vi "MasterAquisitionFile_IOS_Optogenetics_Test.vi"() -> ()   [LabVIEW 2018]
uses:
  <vilib>/vision/driver/IMAQdx.llb/IMAQdx Acquisition Mode.ctl
  <vilib>/vision/driver/IMAQdx.llb/IMAQdx Camera Control Mode.ctl
  <vilib>/userdefined/High Color/IMAQdx.ctl
  <vilib>/vision/driver/IMAQdx.llb/IMAQdx Buffer Number Mode.ctl
  <vilib>/DAQmx/write.llb/DAQmx Write (Analog 1D DBL 1Chan NSamp).vi
  <vilib>/DAQmx/write.llb/DAQmx Write (Digital Bool 1Line 1Point).vi
  <vilib>/DAQmx/read.llb/DAQmx Read (Analog 1D Wfm NChan NSamp).vi
  <vilib>/DAQmx/write.llb/DAQmx Write (Digital 1D Bool 1Chan 1Samp).vi
  <vilib>/DAQmx/create/channels.llb/DAQmx Create Channel (DO-Digital Output).vi
  <vilib>/Waveform/DWDTOps.llb/DWDT Digital to Boolean Array.vi
  <vilib>/DAQmx/create/channels.llb/DAQmx Create Channel (AO-Voltage-Basic).vi
  <vilib>/DAQmx/create/channels.llb/DAQmx Create Channel (CO-Pulse Generation-Frequency).vi
  <vilib>/DAQmx/configure/timing.llb/DAQmx Timing (Implicit).vi
  <vilib>/DAQmx/create/channels.llb/DAQmx Create Channel (AI-Voltage-Basic).vi
  <vilib>/DAQmx/configure/timing.llb/DAQmx Timing (Sample Clock).vi
  <vilib>/DAQmx/configure/trigger.llb/DAQmx Start Trigger (Digital Edge).vi
  <vilib>/DAQmx/miscellaneous.llb/DAQmx Fill In Error Info.vi
  <vilib>/vision/driver/NI_Vision_Acquisition_Software.lvlib
  <resource>/objmgr/imaqdx.rc
  <resource>/objmgr/daqmx.rc
panel:
  out "LED":bool
  out "Auditory":bool
  out "RPad":bool
  out "LPad":bool
  out "Finished":bool
  in  "Solenoids":bool=TRUE
  in  "LED":bool=TRUE
  in  "Sol Stim Parameters":cluster{"Fs":dbl, "Samples":dbl}
  in  "LED Stim Parameters":cluster{"Fs":dbl, "Samples":dbl}
  in  "Sol Duty Cycle (%)":dbl=10.0
  in  "Sol Freq":dbl=1.0
  in  "Sol Dur (s)":dbl=1.0
  in  "LED Duty Cycle (%)":dbl=10.0
  in  "LED Freq":dbl=10.0
  in  "LED Dur (s)":dbl=2.0
  out "Stimulus Order":digitalwaveform[](graph)=[{"t0"=timestamp(0 s since 1904-01-01), "dt"=5e-05, "Y"={"transitions"=[], "data"=array18000000x1[18000000 elements]}}, {"t0"=timestamp(0 s since 1904-01-01), "dt"=5e-05, "Y"={"transitions"=[], "data"=array18000000x1[18000000 elements]}}, {"t0"=timestamp(0 s since 1904-01-01), "dt"=5e-05, "Y"={"transitions"=[], "data"=array18000000x1[18000000 elements]}}, {"t0"=timestamp(0 s since 1904-01-01), "dt"=5e-05, "Y"={"transitions"=[], "data"=array18000000x1[18000000 elements]}}]
  out "Solenoid Stim":digitalwaveform(graph)={"t0"=timestamp(0 s since 1904-01-01), "dt"=5e-05, "Y"={"transitions"=[], "data"=array20000x1[20000 elements]}}
  in  "Trial Offset (s)":dbl=15.0
  in  "Interstim (s)":dbl=30.0
  in  "Right Pad":dbl=1.0
  in  "Left Pad":dbl=1.0
  in  "Auditory":dbl=1.0
  in  "LED":dbl
  out "Dev2 Samples":i32
  out "Dev2 Analog":bool
  in  "Dev2 Analog Channels":string[](array[string])=["LD_BackScatter", "LD_Flow", "Opto_LED", "RPadSol", "AudSol", "Hippocampus", "EMG", "Cortical_RH"]
  out "?":T1(plugin-control)
  out "?":T1(plugin-control)
  out "?":T1(plugin-control)
  out "?":T1(plugin-control)
  in  "stop":bool
  out "CBV Cam":bool
  out "Pupil Cam":bool
  out "Whisk Cam":bool
  out "Web Cam":bool
  out "Dev1 Analog":bool
  out "Web Cam Fs":dbl(knob) scale=0.0..200.0
  out "CBV Cam":dbl(knob) scale=0.0..200.0
  out "Whisk Cam Fs":dbl(knob) scale=0.0..200.0
  out "Last Whisk\nBuffer 2":u32=574
  out "Pupil Cam Fs":dbl(knob) scale=0.0..200.0
  out "Dropped 2":u32(slide) caption="Pupil Cam" scale=0.0..99.0
  in  "Exposure Time (microsec)":string="10000"
  out "Dev1 Samples":i32
  in  "Dev1 Analog Channels":string[](array[string])=["Cortical_LH", "Force_Sensor", "LPadSol", "RPadSol", "AudSol", "Hippocampus", "EMG", "Cortical_RH"]
  in  "Analog Acquisition":cluster{"Analog Fs":u16}={"Analog Fs"=20000} {"Analog Fs" format="%0.0f"}
  in  "Sampling Rates":T2={"CBV Cam Fs"=30, "Whisk Cam Fs"=150, "Web Cam Fs"=15, "Pupil Cam Fs"=30}
  out "Notes Size":i32=7
  out "Notes Reversed":string[](array[string])=["Experimenter", "Animal ID", "Hemisphere", "Solenoid PSI", "Isoflurane time", "Session ID", "Amplifier Gain"]
  out "Notes Array":string[](array[string])=["Amplifier Gain", "Session ID", "Isoflurane time", "Solenoid PSI", "Hemisphere", "Animal ID", "Experimenter"]
  in  "Notes:":T3={"Experimenter"="Kevin", "Animal ID"="T155", "Hemisphere"="Both", "Solenoid PSI"="10", "Isoflurane time"="815", "Session ID"="Imaging Session Four", "Amplifier Gain"="10000", "LED power (mW)"="0"}
  in  "Target Path":path=path "D:/T155/Imaging Session 4 - 7 Nov. 2020" caption="Final Save Location"
  out "Dropped":u32(slide) caption="Whisk Cam" scale=0.0..999.0
  out "Filename":string="201105_15_03_37"
  out "CBV Camera":bool
  out "Time Elapsed (Min)":cluster{dbl, dbl}(slide)={15.0, 0.0} scale=0.0..15.0 scale format="%#_2g"
  in  "Time (min)":dbl(knob)=15.0 min=0.5 max=20.0 step=0.5 scale=0.0..20.0 scale format="%#_2g"
  in  "Temp Path":path=path "D:/LabVIEW Streamed Data" caption="Temporary Path for Streamed Data"
  out "Last CBV\nBuffer":i32=574
  out "Last Whisk\nBuffer":u32=2874
  # "Stimuli"
  # "LPAD"
  # "RPAD"
  # "AUD"
  # "LED"
  # "Ratio"
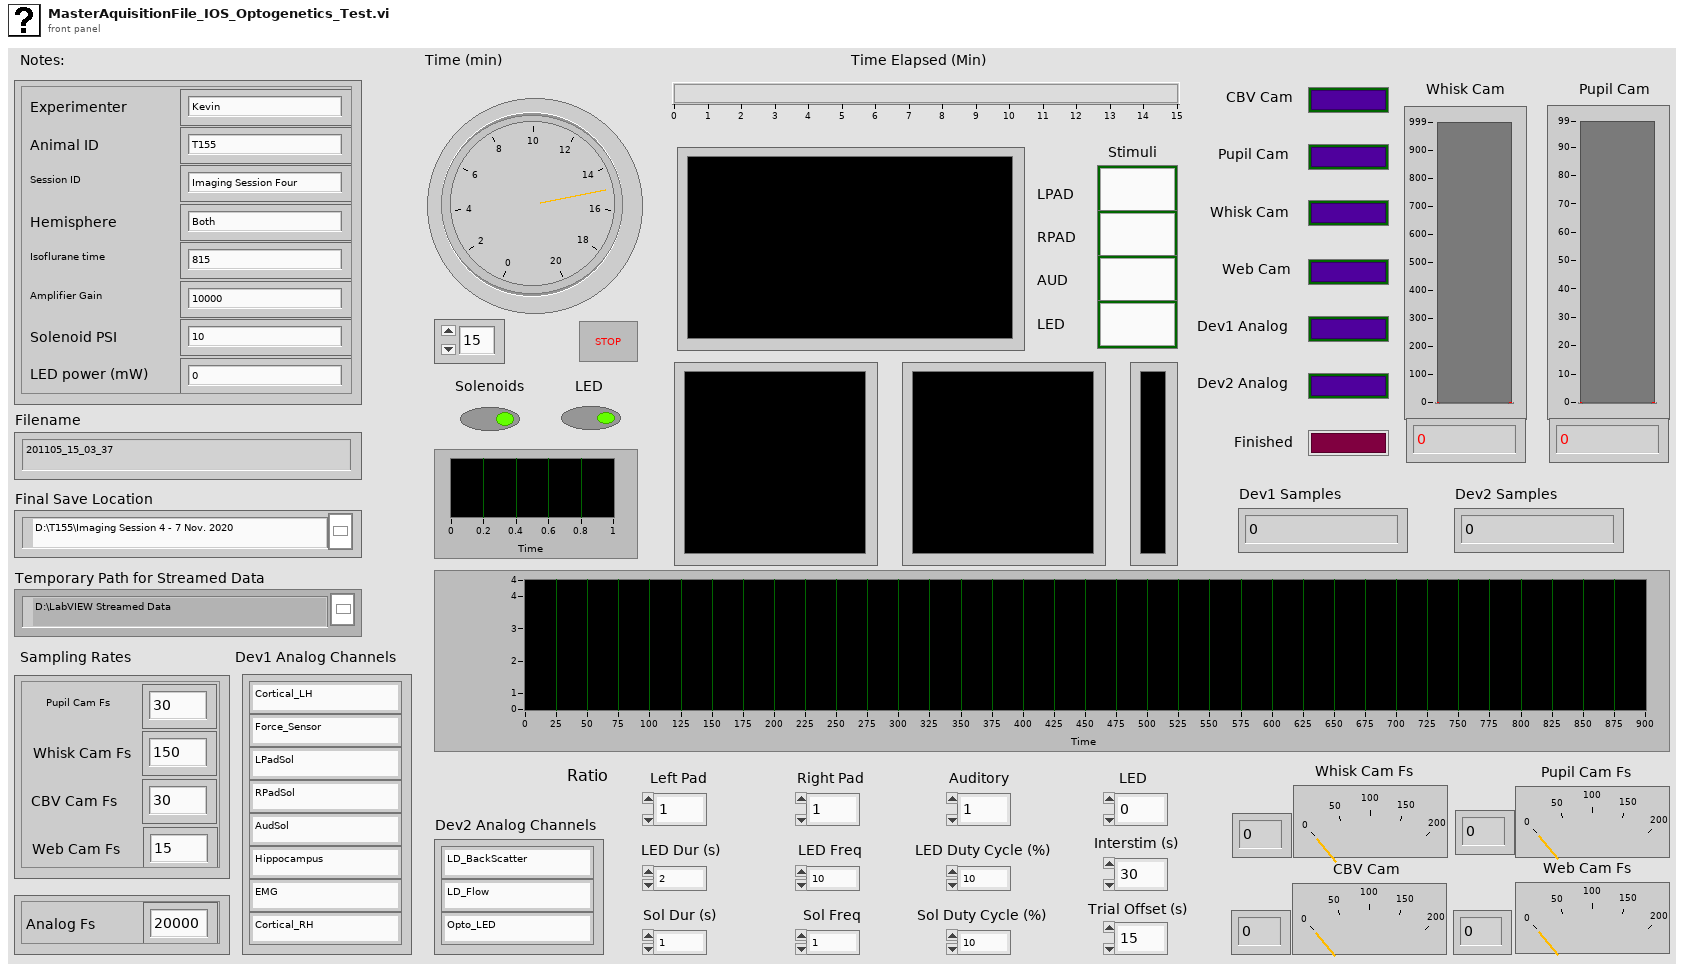
[diagram p1: front panel]
types:
  T1 = typedef "IMAQ Image.ctl" = refnum<image>
  T2 = cluster{"CBV Cam Fs":u16, "Whisk Cam Fs":u16, "Web Cam Fs":u16, "Pupil Cam Fs":u16}
  T3 = cluster{"Experimenter":string, "Animal ID":string, "Hemisphere":string, "Solenoid PSI":string, "Isoflurane time":string, "Session ID":string, "Amplifier Gain":string, "LED power (mW)":string}
  T4 = typedef "IMAQdx.ctl" = refnum<k21>
  T5 = enum16{"open", "open or create", "create or replace", "create", "open (read-only)"}
  T6 = enum16{"open", "replace", "create", "open or create", "replace or create", "replace or create with confirmation"}
  T7 = typedef "Image Type" = u32
  T8 = typedef "NI_Vision_Acquisition_Software.lvlib/IMAQdx Acquisition Mode.ctl" = enum32{"One Shot", "Continuous"}
  T9 = typedef "NI_Vision_Acquisition_Software.lvlib/IMAQdx Camera Control Mode.ctl" = enum32{"Controller", "Listener"}
  T10 = typedef "IMAQ AVI2 Refnum.ctl" = refnum<k20>
  T11 = enum16{"big-endian, network order", "native, host order", "little-endian"}
  T12 = typedef "NI_Vision_Acquisition_Software.lvlib/IMAQdx Buffer Number Mode.ctl" = enum32{"Next", "Last", "Buffer Number", "Every", "Last New"}
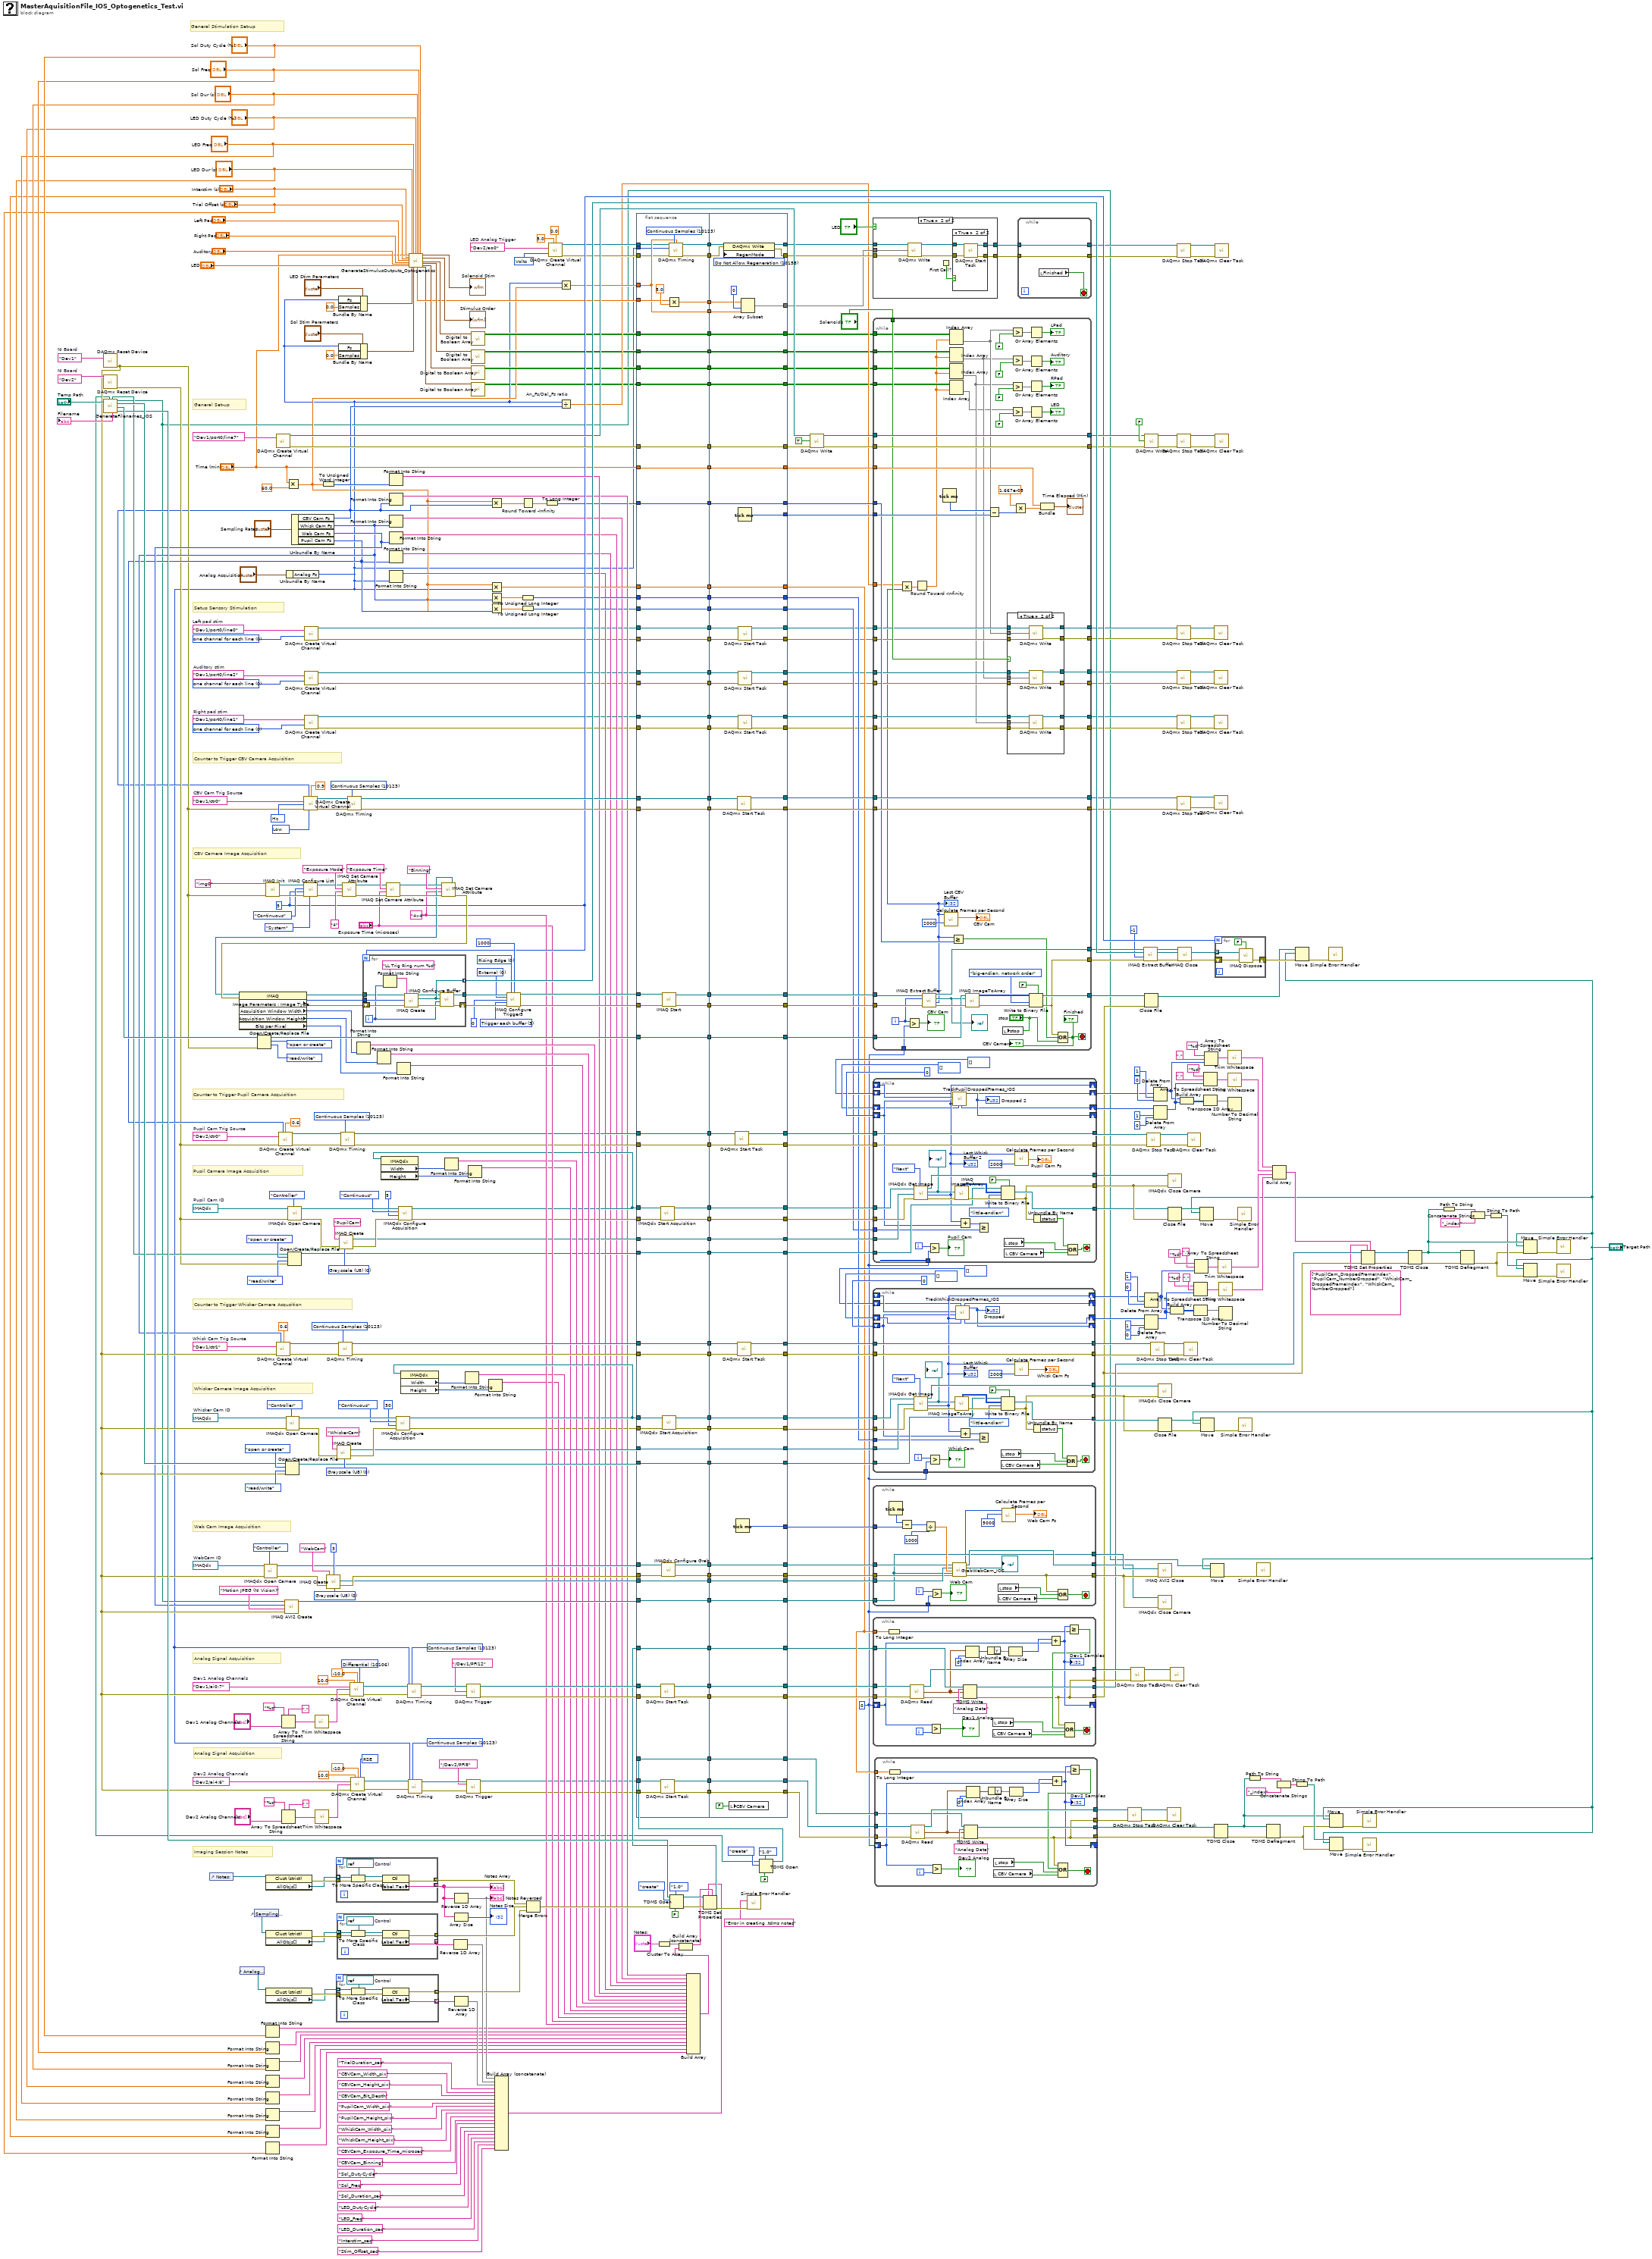
[diagram p0: block diagram]
diagram:
  w159 = tag "Dev2/ai4:6"  # Dev2 Analog Channels
  w357 = tag "Dev1/ai0:7"  # Dev1 Analog Channels
  w360 = T4 "cam0"  # WebCam ID
  w338 = T4 "cam1"  # Whisker Cam ID
  w532 = tag "Dev1/ctr1"  # Whisk Cam Trig Source
  w259 = T4 "cam2"  # Pupil Cam ID
  w264 = tag "Dev2/ctr0"  # Pupil Cam Trig Source
  w506 = tag "Dev1/ctr0"  # CBV Cam Trig Source
  w81 = tag "Dev1/port0/line1"  # Right pad stim
  w79 = tag "Dev1/port0/line0"  # Left pad stim
  w80 = tag "Dev1/port0/line2"  # Auditory stim
  w32 = 0 items=["one channel for each line", "one channel for all lines"] ("line grouping")
  w82 = 0 items=["one channel for each line", "one channel for all lines"] ("line grouping")
  w83 = 0 items=["one channel for each line", "one channel for all lines"] ("line grouping")
  w101 = 10348 items=["Volts"=10348, "From Custom Scale"=10065] ("units")
  w102 = tag "Dev2/ao0"  # LED Analog Trigger
  w163 = 10123 items=["Finite Samples"=10178, "Continuous Samples"=10123, "Hardware Timed Single Point"=12522] ("sample mode")
  w166 = 10083 items=["default"=-1, "RSE"=10083, "NRSE"=10078, "Differential"=10106, "Pseudodifferential"=12529] ("input terminal configuration")
  w182 = tag "Dev2"  # NI Board
  w260 = 10123 items=["Finite Samples"=10178, "Continuous Samples"=10123, "Hardware Timed Single Point"=12522] ("sample mode")
  w267 = T7 0 items=["Grayscale (U8)", "Grayscale (I16)", "Grayscale (SGL)", "Complex (CSG)", "RGB (U32)", "HSL (U32)", "RGB (U64)", "Grayscale (U16)"] ("Image Type")
  w249 = "4x4" ("Attribute Value")
  w118 = 0
  w439 = 10123 items=["Finite Samples"=10178, "Continuous Samples"=10123, "Hardware Timed Single Point"=12522] ("sample mode")
  w442 = 10106 items=["default"=-1, "RSE"=10083, "NRSE"=10078, "Differential"=10106, "Pseudodifferential"=12529] ("input terminal configuration")
  w493 = T7 0 items=["Grayscale (U8)", "Grayscale (I16)", "Grayscale (SGL)", "Complex (CSG)", "RGB (U32)", "HSL (U32)", "RGB (U64)", "Grayscale (U16)"] ("Image Type")
  w513 = u32 0 items=["Rising Edge", "Falling Edge"] ("Trigger Polarity")
  w516 = u32 0 items=["External"=0, "RTSI"=1, "ISO In"=2, "Scaled Encoder"=5] ("Trigger Type")
  w507 = tag "Dev1"  # NI Board
  w508 = 10123 items=["Finite Samples"=10178, "Continuous Samples"=10123, "Hardware Timed Single Point"=12522] ("sample mode")
  w511 = 10373 items=["Hz"=10373] ("units")
  w512 = 10214 items=["High"=10192, "Low"=10214] ("idle state")
  w278 = u32 5 ("Number of Buffers")
  w514 = u32 3 items=["Disabled", "Trigger start of acquisition", "Trigger start of each buffer list", "Trigger each buffer", "Trigger each line (linescan)", "Trigger end of acquisition"] ("Action")
  w528 = 10123 items=["Finite Samples"=10178, "Continuous Samples"=10123, "Hardware Timed Single Point"=12522] ("sample mode")
  w535 = T7 0 items=["Grayscale (U8)", "Grayscale (I16)", "Grayscale (SGL)", "Complex (CSG)", "RGB (U32)", "HSL (U32)", "RGB (U64)", "Grayscale (U16)"] ("Image Type")
  # "General Stimulation Set-up"
  # "Analog Signal Acquisition"
  # "General Set-up"
  # "Pupil Camera Image Acquisition"
  # "Counter to Trigger Pupil Camera Acquisition"
  # "Whisker Camera Image Acquisition"
  # "Imaging Session Notes"
  # "Setup Sensory Stimulation"
  # "CBV Camera Image Acquisition"
  # "Counter to Trigger CBV Camera Acquisition"
  # "Counter to Trigger Whisker Camera Acqusition"
  # "Web Cam Image Acquisition"
  # "Analog Signal Acquisition"
  n1 = call <vilib>:"DAQmx Reset Device.vi"("device in"=w507) -> ("error out"=w152:errorcluster)  [unwired: 14 in]
  n2 = call <vilib>:"DAQmx Reset Device.vi"("device in"=w182) -> ("error out"=w181:errorcluster)  [unwired: 14 in]
  n3 = call "GenerateFilenames_IOS.vi"("path"="Temp Path") -> ("TDMS Path"=w382:path, "Dalsa Path"=w500:path, "Basler Path"=w496:path, "WebCam Path"=w31:path, "Analog file name"=→"Filename":string, "Basler2 Path"=w258:path, "TDMS Path 2"=w120:path)  [unwired: 3 in, 1 out]
  n4 = control-ref of="Notes:"() -> (w387:refnum<vi>)
  n5 = control-ref of="Analog Acquisition"() -> (w365:refnum<vi>)
  n6 = control-ref of="Sampling Rates"() -> (w366:refnum<vi>)
  n7 = Open/Create/Replace File(file path (use dialog)=w500, error in=w152, operation (0:open)=T6."open or create", access (0:read/write)=enum16{"read/write", "read-only", "write-only"}."read/write") -> (refnum out=w443:refnum<file>)  [unwired: 2 in, 2 out]
  n8 = call <vilib>:"IMAQdx Open Camera.vi"("Camera Control Mode"=IMAQdx_Camera_Control_Mode."Controller", "error in"=w152, "Session In"=w360) -> ("error out"=w489:errorcluster, "Session Out"=w487:T4)  [unwired: 7 in]
  n9 = property class="Clust (strict)"(reference=w387) -> (error out=w390:errorcluster, "AllObjs[]"=w285:refnum<vi>[])  [unwired: 1 in, 1 out]
  n10 = property class="Clust (strict)"(reference=w366) -> (error out=w385:errorcluster, "AllObjs[]"=w286:refnum<vi>[])  [unwired: 1 in, 1 out]
  n11 = property class="Clust (strict)"(reference=w365) -> (error out=w364:errorcluster, "AllObjs[]"=w284:refnum<vi>[])  [unwired: 1 in, 1 out]
  n12 = call <vilib>:"IMAQ Init.vi"("error in (no error)"=w152, "Interface Name"="img0") -> ("error out"=w526:errorcluster, "IMAQ Session Out"=w527:refnum<k11>)  [unwired: 8 out]
  n13 = Format Into String("Sol Duty Cycle (%)") -> (resulting string=w20:string)  [unwired: 3 in, 1 out]
  n14 = Format Into String("Sol Freq") -> (resulting string=w19:string)  [unwired: 3 in, 1 out]
  n15 = Format Into String("Sol Dur (s)") -> (resulting string=w18:string)  [unwired: 3 in, 1 out]
  n16 = Format Into String("LED Duty Cycle (%)") -> (resulting string=w17:string)  [unwired: 3 in, 1 out]
  n17 = Format Into String("LED Freq") -> (resulting string=w16:string)  [unwired: 3 in, 1 out]
  n18 = Format Into String("LED Dur (s)") -> (resulting string=w15:string)  [unwired: 3 in, 1 out]
  n19 = Format Into String("Interstim (s)") -> (resulting string=w14:string)  [unwired: 3 in, 1 out]
  n20 = Format Into String("Trial Offset (s)") -> (resulting string=w13:string)  [unwired: 3 in, 1 out]
  n21 = call-poly <vilib>:"DAQmx Create Virtual Channel.vi"("lines"=tag "Dev1/port0/line7") -> ("task out"=w316:refnum<k21>, "error out"=w319:errorcluster)  [unwired: 13 in]
  n22 = Array To Spreadsheet String(delimiter (Tab)=",", array="Dev1 Analog Channels", 3:"%s" ("format string")) -> (spreadsheet string=w354:string)
  n23 = Array To Spreadsheet String(delimiter (Tab)=",", array="Dev2 Analog Channels", 3:"%s" ("format string")) -> (spreadsheet string=w156:string)
  n24 = Open/Create/Replace File(file path (use dialog)=w496, error in=w152, operation (0:open)=T6."open or create", access (0:read/write)=enum16{"read/write", "read-only", "write-only"}."read/write") -> (refnum out=w461:refnum<file>)  [unwired: 2 in, 2 out]
  n25 = Unbundle By Name("Analog Acquisition") -> ("Analog Fs"=w29:u16)
  n26 = call <vilib>:"IMAQdx Open Camera.vi"("Camera Control Mode"=IMAQdx_Camera_Control_Mode."Controller", "error in"=w152, "Session In"=w338) -> ("error out"=w538:errorcluster, "Session Out"=w541:T4)  [unwired: 7 in]
  n27 = Multiply(x="Time (min)", y=60.0) -> (x*y=w33:dbl)
  n28 = Open/Create/Replace File(file path (use dialog)=w258, error in=w181, operation (0:open)=T6."open or create", access (0:read/write)=enum16{"read/write", "read-only", "write-only"}."read/write") -> (refnum out=w239:refnum<file>)  [unwired: 2 in, 2 out]
  n29 = call <vilib>:"IMAQdx Open Camera.vi"("Camera Control Mode"=IMAQdx_Camera_Control_Mode."Controller", "error in"=w181, "Session In"=w259) -> ("error out"=w270:errorcluster, "Session Out"=w273:T4)  [unwired: 7 in]
  n30 = Unbundle By Name("Sampling Rates") -> ("CBV Cam Fs"=w84:u16, "Whisk Cam Fs"=w221:u16, "Web Cam Fs"=w359:u16, "Pupil Cam Fs"=w215:u16)
  n31 = call-poly <vilib>:"DAQmx Create Virtual Channel.vi"("frequency"=w221, "duty cycle"=0.6, "counter"=w532, "error in"=w152) -> ("task out"=w530:refnum<k21>, "error out"=w529:errorcluster)  [unwired: 10 in]
  n32 = call-poly <vilib>:"DAQmx Create Virtual Channel.vi"("frequency"=w215, "duty cycle"=0.6, "counter"=w264, "error in"=w181) -> ("task out"=w262:refnum<k21>, "error out"=w261:errorcluster)  [unwired: 10 in]
  n33 = call "IMAQ AVI2 Create"("error in (no error)"=w152, "Codec"="Motion JPEG (NI Vision)", "Frames Per Second"=w359, "AVI Path"=w31) -> ("AVI Refnum"=w479:T10)  [unwired: 6 in, 1 out]
  n34 = call-poly <vilib>:"DAQmx Create Virtual Channel.vi"("frequency"=w84, "duty cycle"=0.9, "counter"=w506, "units"=w511, "error in"=w152, "idle state"=w512) -> ("task out"=w510:refnum<k21>, "error out"=w509:errorcluster)  [unwired: 8 in]
  n35 = call <vilib>:"IMAQ Configure List.vi"("Memory Location"=enum16{"System", "Onboard"}."System", "error in (no error)"=w526, "Number of buffers"=w278, "Continuous?"=enum16{"One-Shot", "Continuous"}."Continuous" ("Continuous ?"), "IMAQ Session In"=w527) -> ("error out"=w299:errorcluster, "IMAQ Session Out"=w295:refnum<k11>)  [unwired: 1 in, 4 out]
  n36 = call-poly <vilib>:"DAQmx Create Virtual Channel.vi"("lines"=w79, "line grouping"=w32) -> ("task out"=w60:refnum<k21>, "error out"=w58:errorcluster)  [unwired: 12 in]
  n37 = call-poly <vilib>:"DAQmx Create Virtual Channel.vi"("lines"=w80, "line grouping"=w82) -> ("task out"=w56:refnum<k21>, "error out"=w54:errorcluster)  [unwired: 12 in]
  n38 = call-poly <vilib>:"DAQmx Create Virtual Channel.vi"("lines"=w81, "line grouping"=w83) -> ("task out"=w52:refnum<k21>, "error out"=w50:errorcluster)  [unwired: 12 in]
  n39 = call <vilib>:"Trim Whitespace.vi"("string"=w354) -> ("trimmed string"=w353:string)  [unwired: 1 in]
  n40 = call <vilib>:"Trim Whitespace.vi"("string"=w156) -> ("trimmed string"=w155:string)  [unwired: 1 in]
  n41 = To Unsigned Word Integer(number=w33) -> (unsigned 16bit integer=w349:u16)
  n42 = call "IMAQ Create"("Border Size"=3, "Image Name"="WebCam", "Image Type"=w493, "error in (no error)"=w489) -> ("New Image"=w486:T1, "error out"=w488:errorcluster)  [unwired: 1 in]
  n43 = for {
    tunnel: [w547] -> w389 mode=indexing
    tunnel: w390 -> [w546]
    tunnel: [w544] -> w373 mode=indexing
    tunnel: w285 -> [w543] mode=indexing
    w548 = refnum<vi> refnum  # Control
    n44 = To More Specific Class(target class=w548, reference=w543, error in=w546) -> (specific class reference=w549:refnum<vi>, error out=w545:errorcluster)
    n45 = property class="Ctl"(reference=w549, error in=w545) -> (error out=w544:errorcluster, "Label.Text"=w547:string)  [unwired: 1 out]
  }
  "Notes Array" <- w389
  n46 = for {
    tunnel: [w554] -> w362 mode=indexing
    tunnel: w364 -> [w553]
    tunnel: [w551] -> w363 mode=indexing
    tunnel: w284 -> [w550] mode=indexing
    w555 = refnum<vi> refnum  # Control
    n47 = To More Specific Class(target class=w555, reference=w550, error in=w553) -> (specific class reference=w556:refnum<vi>, error out=w552:errorcluster)
    n48 = property class="Ctl"(reference=w556, error in=w552) -> (error out=w551:errorcluster, "Label.Text"=w554:string)  [unwired: 1 out]
  }
  n49 = call "IMAQ Create"("Image Name"="WhiskerCam", "Image Type"=w535, "error in (no error)"=w538) -> ("New Image"=w336:T1, "error out"=w536:errorcluster)  [unwired: 2 in]
  n50 = for {
    tunnel: [w561] -> w386 mode=indexing
    tunnel: w385 -> [w560]
    tunnel: [w558] -> w372 mode=indexing
    tunnel: w286 -> [w557] mode=indexing
    w562 = refnum<vi> refnum  # Control
    n51 = To More Specific Class(target class=w562, reference=w557, error in=w560) -> (specific class reference=w563:refnum<vi>, error out=w559:errorcluster)
    n52 = property class="Ctl"(reference=w563, error in=w559) -> (error out=w558:errorcluster, "Label.Text"=w561:string)  [unwired: 1 out]
  }
  n53 = Bundle By Name(cluster="LED Stim Parameters", "Fs"=w29, "Samples"=0.0) -> (w107:cluster{"Fs":dbl, "Samples":dbl})
  n54 = Bundle By Name(cluster="Sol Stim Parameters", "Fs"=w29, "Samples"=0.0) -> (w108:cluster{"Fs":dbl, "Samples":dbl})
  n55 = call-poly <vilib>:"DAQmx Timing.vi"("task/channels in"=w530, "sample mode"=w528, "error in"=w529) -> ("task out"=w424:refnum<k21>, "error out"=w422:errorcluster)  [unwired: 11 in]
  n56 = call "IMAQ Create"("Image Name"="PupilCam", "Image Type"=w267, "error in (no error)"=w270) -> ("New Image"=w224:T1, "error out"=w268:errorcluster)  [unwired: 2 in]
  n57 = call-poly <vilib>:"DAQmx Timing.vi"("task/channels in"=w262, "sample mode"=w260, "error in"=w261) -> ("task out"=w237:refnum<k21>, "error out"=w235:errorcluster)  [unwired: 11 in]
  n58 = call <vilib>:"IMAQ Set Camera Attribute.vi"("error in (no error)"=w299, "Attribute Value"="4", "Camera Attribute"="Exposure Mode", "IMAQ Session In"=w295) -> ("error out"=w298:errorcluster, "IMAQ Session Out"=w294:refnum<k11>)  [unwired: 4 in]
  n59 = call-poly <vilib>:"DAQmx Timing.vi"("task/channels in"=w510, "sample mode"=w508, "error in"=w509) -> ("task out"=w428:refnum<k21>, "error out"=w426:errorcluster)  [unwired: 11 in]
  n60 = call-poly <vilib>:"DAQmx Create Virtual Channel.vi"("maximum value"=10.0, "minimum value"=-10.0, "input terminal configuration"=w442, "physical channels"=w357, "name to assign"=w353, "error in"=w152) -> ("task out"=w441:refnum<k21>, "error out"=w440:errorcluster)  [unwired: 8 in]
  n61 = call-poly <vilib>:"DAQmx Create Virtual Channel.vi"("maximum value"=10.0, "minimum value"=-10.0, "input terminal configuration"=w166, "physical channels"=w159, "name to assign"=w155, "error in"=w152) -> ("task out"=w165:refnum<k21>, "error out"=w164:errorcluster)  [unwired: 8 in]
  n62 = call <vilib>:"IMAQ Set Camera Attribute.vi"("error in (no error)"=w298, "Attribute Value"="Exposure Time (microsec)", "Camera Attribute"="Exposure Time", "IMAQ Session In"=w294) -> ("error out"=w297:errorcluster, "IMAQ Session Out"=w293:refnum<k11>)  [unwired: 4 in]
  n63 = Format Into String(w349) -> (resulting string=w351:string)  [unwired: 3 in, 1 out]
  n64 = Format Into String(w84) -> (resulting string=w219:string)  [unwired: 3 in, 1 out]
  n65 = Format Into String(w221) -> (resulting string=w218:string)  [unwired: 3 in, 1 out]
  n66 = Format Into String(w359) -> (resulting string=w217:string)  [unwired: 3 in, 1 out]
  n67 = Format Into String(w215) -> (resulting string=w168:string)  [unwired: 3 in, 1 out]
  n68 = Format Into String(w29) -> (resulting string=w167:string)  [unwired: 3 in, 1 out]
  n69 = call <vilib>:"IMAQdx Configure Acquisition.vi"("error in"=w536, "Number of Buffers"=u32 50, "Continuous?"=IMAQdx_Acquisition_Mode."Continuous", "Session In"=w541) -> ("error out"=w183:errorcluster, "Session Out"=w337:T4)  [unwired: 6 in]
  n70 = call <vilib>:"IMAQdx Configure Acquisition.vi"("error in"=w268, "Number of Buffers"=u32 5, "Continuous?"=IMAQdx_Acquisition_Mode."Continuous", "Session In"=w273) -> ("error out"=w241:errorcluster, "Session Out"=w225:T4)  [unwired: 6 in]
  n71 = property class="IMAQdx"(reference=w225) -> ("Width"=w257:u32, "Height"=w256:u32)  [unwired: 1 in, 2 out]
  n72 = property class="IMAQdx"(reference=w337) -> ("Width"=w348:u32, "Height"=w347:u32)  [unwired: 1 in, 2 out]
  n73 = call-poly <vilib>:"DAQmx Timing.vi"("task/channels in"=w441, "sample mode"=w439, "rate"=w29, "error in"=w440) -> ("task out"=w282:refnum<k21>, "error out"=w438:errorcluster)  [unwired: 10 in]
  n74 = call-poly <vilib>:"DAQmx Timing.vi"("task/channels in"=w165, "sample mode"=w163, "rate"=w29, "error in"=w164) -> ("task out"=w153:refnum<k21>, "error out"=w162:errorcluster)  [unwired: 10 in]
  n75 = call "GenerateStimulusOutputs_Optogenetics.vi"("Trial duration (min)"="Time (min)", "Rest duration(s)"="Interstim (s)", "trial offset (s)"="Trial Offset (s)", "Left Pad"="Left Pad", "Right Pad"="Right Pad", "Auditory"="Auditory", "LED"="LED", "LED Stim Duration (s)"="LED Dur (s)", "LED Stim Parameters"=w107, "LED Frequency"="LED Freq", "Sol Stim Parameters"=w108, "LED duty cycle (%)"="LED Duty Cycle (%)", "Sol Stim Duration (s)"="Sol Dur (s)", "Sol Frequency"="Sol Freq", "Sol Duty Cycle (%)"="Sol Duty Cycle (%)") -> ("Double LED Out"=w95:dbl[], "Solenoid Stim Waveforms"=→"Solenoid Stim":digitalwaveform, "Stimulus Digital Outputs"=→"Stimulus Order":digitalwaveform[], "Left Pad Out"=w113:digitalwaveform, "Auditory Out"=w112:digitalwaveform, "Right Pad Out"=w111:digitalwaveform, "LED Out"=w2:digitalwaveform)  [unwired: 6 in]
  n76 = call <vilib>:"IMAQ Set Camera Attribute.vi"("error in (no error)"=w297, "Attribute Value"=w249, "Camera Attribute"="Binning", "IMAQ Session In"=w293) -> ("error out"=w296:errorcluster, "IMAQ Session Out"=w292:refnum<k11>)  [unwired: 4 in]
  n77 = property class="IMAQ"(reference=w292, error in=w296) -> (reference out=w306:refnum<k11>, error out=w305:errorcluster, "Image Parameters : Image Type"=w522:u32, "Acquisition Window Width"=w346:u32, "Acquisition Window Height"=w345:u32, "Bits per Pixel"=w344:u32)
  n78 = Format Into String(w346) -> (resulting string=w343:string)  [unwired: 3 in, 1 out]
  n79 = for {
    N: w278 -> [_]
    tunnel: [w573] -> w518
    tunnel: w522 -> [w571]
    shift-right: [w572] -> w517
    shift-left: w305 -> [w570]
    tunnel: [w565] -> w519 mode=indexing
    tunnel: w306 -> [w564]
    i -> [w566]
    n80 = Format Into String(format string="LL Trig Ring num %d", w566) -> (resulting string=w568:string)  [unwired: 2 in, 1 out]
    n81 = call "IMAQ Create"("Image Name"=w568, "Image Type"=w571, "error in (no error)"=w570) -> ("New Image"=w565:T1, "error out"=w569:errorcluster)  [unwired: 1 in, 1 out]
    n82 = call <vilib>:"IMAQ Configure Buffer.vi"("error in (no error)"=w569, "Buffer Number"=w566, "Image In"=w565, "IMAQ Session In"=w564) -> ("error out"=w572:errorcluster, "IMAQ Session Out"=w573:refnum<k11>)  [unwired: 2 in, 4 out]
  }
  n83 = Format Into String(w345) -> (resulting string=w279:string)  [unwired: 3 in, 1 out]
  n84 = Format Into String(w344) -> (resulting string=w342:string)  [unwired: 3 in, 1 out]
  n85 = Format Into String(w257) -> (resulting string=w244:string)  [unwired: 3 in, 1 out]
  n86 = Reverse 1D Array(array=w386) -> (reversed array=w376:string[])
  n87 = Reverse 1D Array(array=w389) -> (reversed array=w283:string[])
  "Notes Reversed" <- w283
  n88 = Array Size(array=w389) -> (size(s)=→"Notes Size":i32)
  n89 = Reverse 1D Array(array=w362) -> (reversed array=w361:string[])
  n90 = Format Into String(w348) -> (resulting string=w246:string)  [unwired: 3 in, 1 out]
  n91 = call-poly <vilib>:"DAQmx Trigger.vi"("task/channels in"=w282, "source"=tag "/Dev1/PFI12", "error in"=w438) -> ("task out"=w437:refnum<k21>, "error out"=w436:errorcluster)  [unwired: 11 in]
  n92 = call-poly <vilib>:"DAQmx Trigger.vi"("task/channels in"=w153, "source"=tag "/Dev2/PFI8", "error in"=w162) -> ("task out"=w151:refnum<k21>, "error out"=w150:errorcluster)  [unwired: 11 in]
  n93 = Format Into String(w256) -> (resulting string=w245:string)  [unwired: 3 in, 1 out]
  n94 = call-poly <vilib>:"Digital to Boolean Array.vi"("digital waveform"=w113) -> ("boolean array"=w46:bool[][])  [unwired: 9 in, 1 out]
  n95 = call-poly <vilib>:"Digital to Boolean Array.vi"("digital waveform"=w112) -> ("boolean array"=w43:bool[][])  [unwired: 9 in, 1 out]
  n96 = call-poly <vilib>:"Digital to Boolean Array.vi"("digital waveform"=w111) -> ("boolean array"=w40:bool[][])  [unwired: 9 in, 1 out]
  n97 = call-poly <vilib>:"Digital to Boolean Array.vi"("digital waveform"=w2) -> ("boolean array"=w1:bool[][])  [unwired: 9 in, 1 out]
  n98 = Format Into String(w347) -> (resulting string=w247:string)  [unwired: 3 in, 1 out]
  n99 = Multiply(x=w33, y=w84) -> (x*y=w498:dbl)
  n100 = Multiply(x=w33, y=w29) -> (x*y=w325:dbl)
  n101 = Multiply(x=w221, y=w33) -> (x*y=w280:dbl)
  n102 = Multiply(x=w215, y=w33) -> (x*y=w220:dbl)
  n103 = Build Array (concatenate)(w283, w376, w361, "TrialDuration_sec", "CBVCam_Width_pix", "CBVCam_Height_pix", "CBVCam_Bit_Depth", "PupilCam_Width_pix", "PupilCam_Height_pix", "WhiskCam_Width_pix", "WhiskCam_Height_pix", "CBVCam_Exposure_Time_microsec" ("element"), "CBVCam_Binning" ("element"), "Sol_DutyCycle", "Sol_Freq", "Sol_Duration_sec", "LED_DutyCycle", "LED_Freq", "LED_Duration_sec", "Interstim_sec", "Stim_Offset_sec") -> (w275:string[])
  n104 = call <vilib>:"IMAQ Configure Trigger3.vi"("IMAQ Session In"=w518, "Polarity"=w513, "Frame timeout (ms)"=u32 1000 ("Frame Timeout (ms)"), "Type"=w516, "Line Number"=u32 0 ("Trigger Line Number"), "Action"=w514, "error in (no error)"=w517) -> ("IMAQ Session Out"=w460:refnum<k11>, "error out"=w459:errorcluster)  [unwired: 2 in, 5 out]
  n105 = To Unsigned Long Integer(number=w280) -> (unsigned 32bit integer=w323:u32)
  n106 = To Unsigned Long Integer(number=w220) -> (unsigned 32bit integer=w216:u32)
  n107 = Round Toward -Infinity(1:w498) -> (0:w497:dbl)
  n108 = Merge Errors(w373, w372, w363) -> (w371:errorcluster)
  n109 = To Long Integer(number=w497) -> (32bit integer=w184:i32)
  n110 = call-poly <vilib>:"DAQmx Create Virtual Channel.vi"("maximum value"=5.0, "minimum value"=0.0, "physical channels"=w102, "units"=w101) -> ("task out"=w91:refnum<k21>, "error out"=w88:errorcluster)  [unwired: 10 in]
  n111 = Multiply(x=w29, y=w33) -> (x*y=w93:dbl)
  n112 = Divide "An_Fs/Dal_Fs ratio"(x=w29, y=w84) -> (x/y=w47:dbl)
  n113 = flat-sequence {
    tunnel: w488 -> [w638]
    tunnel: w487 -> [w637]
    tunnel: w486 -> [w636]
    tunnel: [w636] -> w485
    tunnel: [w635] -> w483
    tunnel: [w634] -> w481
    tunnel: w479 -> [w633]
    tunnel: [w633] -> w478
    tunnel: w337 -> [w632]
    tunnel: w183 -> [w631]
    tunnel: [w630] -> w468
    tunnel: [w629] -> w466
    tunnel: [w628] -> w464
    tunnel: w336 -> [w628]
    tunnel: [w627] -> w462
    tunnel: w461 -> [w627]
    tunnel: w460 -> [w626]
    tunnel: w459 -> [w625]
    tunnel: [w624] -> w457
    tunnel: [w623] -> w455
    tunnel: w184 -> [w622]
    tunnel: [w622] -> w449
    tunnel: "Time (min)" -> [w621]
    tunnel: [w621] -> w446
    tunnel: [w620] -> w444
    tunnel: w443 -> [w620]
    tunnel: w437 -> [w619]
    tunnel: w436 -> [w618]
    tunnel: [w617] -> w435
    tunnel: [w616] -> w434
    tunnel: [w615] -> w430
    tunnel: w374 -> [w615]
    tunnel: w428 -> [w614]
    tunnel: [w614] -> w427
    tunnel: w426 -> [w613]
    tunnel: [w613] -> w425
    tunnel: w424 -> [w612]
    tunnel: [w612] -> w423
    tunnel: w422 -> [w611]
    tunnel: [w611] -> w421
    tunnel: w325 -> [w610]
    tunnel: [w610] -> w324
    tunnel: w323 -> [w609]
    tunnel: [w609] -> w322
    tunnel: w319 -> [w608]
    tunnel: [w608] -> w318
    tunnel: [w601] -> w243
    tunnel: w225 -> [w602]
    tunnel: [w599] -> w242
    tunnel: w241 -> [w600]
    tunnel: [w607] -> w240
    tunnel: w239 -> [w607]
    tunnel: [w606] -> w238
    tunnel: w237 -> [w606]
    tunnel: [w605] -> w236
    tunnel: w235 -> [w605]
    tunnel: w224 -> [w604]
    tunnel: [w604] -> w223
    tunnel: w216 -> [w603]
    tunnel: [w603] -> w214
    tunnel: w151 -> [w598]
    tunnel: w150 -> [w597]
    tunnel: [w596] -> w149
    tunnel: [w595] -> w148
    tunnel: w123 -> [w594]
    tunnel: [w594] -> w122
    tunnel: w95 -> [w591]
    tunnel: [w590] -> w94
    tunnel: w93 -> [w589]
    tunnel: [w589] -> w92
    tunnel: w91 -> [w588]
    tunnel: [w587] -> w90
    tunnel: [w586] -> w89
    tunnel: w88 -> [w585]
    tunnel: w29 -> [w584]
    tunnel: w60 -> [w583]
    tunnel: [w583] -> w59
    tunnel: w58 -> [w582]
    tunnel: [w582] -> w57
    tunnel: w56 -> [w581]
    tunnel: [w581] -> w55
    tunnel: w54 -> [w580]
    tunnel: [w580] -> w53
    tunnel: w52 -> [w579]
    tunnel: [w579] -> w51
    tunnel: w50 -> [w578]
    tunnel: [w578] -> w49
    tunnel: w46 -> [w577]
    tunnel: [w577] -> w45
    tunnel: w43 -> [w576]
    tunnel: [w576] -> w42
    tunnel: w40 -> [w575]
    tunnel: [w575] -> w39
    tunnel: w1 -> [w574]
    tunnel: [w574] -> w4
    tunnel: [w705] -> w490
    tunnel: w485 -> [w704]
    tunnel: [w704] -> w484
    tunnel: w483 -> [w703]
    tunnel: [w703] -> w482
    tunnel: w481 -> [w702]
    tunnel: [w702] -> w480
    tunnel: w478 -> [w701]
    tunnel: [w701] -> w477
    tunnel: [w683] -> w474
    tunnel: [w682] -> w472
    tunnel: [w700] -> w469
    tunnel: w468 -> [w700]
    tunnel: [w699] -> w467
    tunnel: w466 -> [w699]
    tunnel: [w698] -> w465
    tunnel: w464 -> [w698]
    tunnel: [w697] -> w463
    tunnel: w462 -> [w697]
    tunnel: [w696] -> w458
    tunnel: w457 -> [w696]
    tunnel: [w695] -> w456
    tunnel: w455 -> [w695]
    tunnel: [w687] -> w453
    tunnel: [w686] -> w451
    tunnel: [w694] -> w450
    tunnel: w449 -> [w693]
    tunnel: [w693] -> w448
    tunnel: [w692] -> w447
    tunnel: w446 -> [w692]
    tunnel: [w691] -> w445
    tunnel: w444 -> [w691]
    tunnel: [w690] -> w432
    tunnel: w435 -> [w690]
    tunnel: [w689] -> w433
    tunnel: w434 -> [w689]
    tunnel: [w688] -> w146
    tunnel: w430 -> [w688]
    tunnel: w427 -> [w685]
    tunnel: w425 -> [w684]
    tunnel: w423 -> [w681]
    tunnel: w421 -> [w680]
    tunnel: w324 -> [w679]
    tunnel: [w679] -> w147
    tunnel: w322 -> [w678]
    tunnel: [w678] -> w213
    tunnel: w318 -> [w677]
    tunnel: [w677] -> w317
    tunnel: w243 -> [w675]
    tunnel: w242 -> [w674]
    tunnel: w240 -> [w673]
    tunnel: w238 -> [w670]
    tunnel: w236 -> [w669]
    tunnel: [w667] -> w231
    tunnel: [w668] -> w230
    tunnel: [w675] -> w229
    tunnel: [w674] -> w228
    tunnel: [w673] -> w227
    tunnel: [w672] -> w222
    tunnel: w223 -> [w672]
    tunnel: [w671] -> w212
    tunnel: w214 -> [w671]
    tunnel: [w666] -> w144
    tunnel: w149 -> [w666]
    tunnel: [w665] -> w145
    tunnel: w148 -> [w665]
    tunnel: [w664] -> w121
    tunnel: w122 -> [w664]
    tunnel: w94 -> [w661]
    tunnel: w92 -> [w660]
    tunnel: w90 -> [w659]
    tunnel: w89 -> [w658]
    tunnel: [w657] -> w87
    tunnel: [w656] -> w86
    tunnel: [w655] -> w85
    tunnel: [w654] -> w66
    tunnel: [w653] -> w65
    tunnel: [w652] -> w64
    tunnel: [w651] -> w63
    tunnel: [w650] -> w62
    tunnel: [w649] -> w61
    tunnel: w59 -> [w648]
    tunnel: w57 -> [w647]
    tunnel: w55 -> [w646]
    tunnel: w53 -> [w645]
    tunnel: w51 -> [w644]
    tunnel: w49 -> [w643]
    tunnel: w45 -> [w642]
    tunnel: [w642] -> w44
    tunnel: w42 -> [w641]
    tunnel: [w641] -> w41
    tunnel: w39 -> [w640]
    tunnel: [w640] -> w38
    tunnel: w4 -> [w639]
    tunnel: [w639] -> w3
    frame #0 {
      w593 = 10123 items=["Finite Samples"=10178, "Continuous Samples"=10123, "Hardware Timed Single Point"=12522] ("sample mode")
      n114 = call <vilib>:"IMAQdx Start Acquisition.vi"("error in"=w600, "Session In"=w602) -> ("error out"=w599:errorcluster, "Session Out"=w601:T4)  [unwired: 8 in]
      n115 = call <vilib>:"DAQmx Start Task.vi"("task/channels in"=w619, "error in"=w618) -> ("task out"=w617:refnum<k21>, "error out"=w616:errorcluster)  [unwired: 12 in]
      n116 = call <vilib>:"DAQmx Start Task.vi"("task/channels in"=w598, "error in"=w597) -> ("task out"=w595:refnum<k21>, "error out"=w596:errorcluster)  [unwired: 12 in]
      n117 = call <vilib>:"IMAQdx Configure Grab.vi"("error in"=w638, "Session In"=w637) -> ("error out"=w634:errorcluster, "Session Out"=w635:T4)  [unwired: 8 in]
      n118 = call <vilib>:"IMAQ Start.vi"("error in (no error)"=w625, "IMAQ Session In"=w626) -> ("error out"=w623:errorcluster, "IMAQ Session Out"=w624:refnum<k11>)  [unwired: 8 out]
      n119 = call <vilib>:"IMAQdx Start Acquisition.vi"("error in"=w631, "Session In"=w632) -> ("error out"=w629:errorcluster, "Session Out"=w630:T4)  [unwired: 8 in]
      n120 = Multiply(x=w591, y=5.0) -> (x*y=w590:dbl[])
      n121 = call-poly <vilib>:"DAQmx Timing.vi"("task/channels in"=w588, "sample mode"=w593, "samples per channel"=w589, "rate"=w584, "error in"=w585) -> ("task out"=w587:refnum<k21>, "error out"=w586:errorcluster)  [unwired: 9 in]
    }
    frame #1 {
      w662 = 10158 items=["Allow Regeneration"=10097, "Do Not Allow Regeneration"=10158] ("RegenMode")
      n122 = property class="DAQmx Write"(reference=w659, error in=w658, "RegenMode"=w662) -> (reference out=w657:refnum<k21>, error out=w656:errorcluster)
      n123 = local write "CBV Camera"(FALSE ("Finished Acquiring")) -> ()
      n124 = call <vilib>:"DAQmx Start Task.vi"("task/channels in"=w670, "error in"=w669) -> ("task out"=w667:refnum<k21>, "error out"=w668:errorcluster)  [unwired: 12 in]
      n125 = Tick Count (ms)() -> (millisecond timer value=w705:u32)
      n126 = call <vilib>:"DAQmx Start Task.vi"("task/channels in"=w685, "error in"=w684) -> ("task out"=w687:refnum<k21>, "error out"=w686:errorcluster)  [unwired: 12 in]
      n127 = call <vilib>:"DAQmx Start Task.vi"("task/channels in"=w681, "error in"=w680) -> ("task out"=w683:refnum<k21>, "error out"=w682:errorcluster)  [unwired: 12 in]
      n128 = Tick Count (ms)() -> (millisecond timer value=w694:u32)
      n129 = call <vilib>:"DAQmx Start Task.vi"("task/channels in"=w648, "error in"=w647) -> ("task out"=w649:refnum<k21>, "error out"=w650:errorcluster)  [unwired: 12 in]
      n130 = call <vilib>:"DAQmx Start Task.vi"("task/channels in"=w646, "error in"=w645) -> ("task out"=w651:refnum<k21>, "error out"=w652:errorcluster)  [unwired: 12 in]
      n131 = call <vilib>:"DAQmx Start Task.vi"("task/channels in"=w644, "error in"=w643) -> ("task out"=w653:refnum<k21>, "error out"=w654:errorcluster)  [unwired: 12 in]
      n132 = Array Subset(array=w661, index=0, length=w660) -> (w655:dbl[])
    }
  }
  n133 = Cluster To Array(cluster="Notes:") -> (array=w383:string[])
  n134 = TDMS Open(6:FALSE ("disable buffering? (T)"), 7:enum16{"1.0", "2.0"}."1.0" ("file format version (2.0)"), 8:w371, 10:T5."create" ("operation (0:open)"), 11:w382) -> (0:w377:errorcluster, 3:w378:refnum<k34>)  [unwired: 2 in]
  n135 = Build Array(w219, w218, w217, w168, w167, w351, w343, w279, w342, w244, w245, w246, w247, "Exposure Time (microsec)", w249, w20, w19, w18, w17, w16, w15, w14, w13) -> (w358:string[])
  n136 = Build Array (concatenate)(w383, w358) -> (w375:string[])
  n137 = TDMS Set Properties(5:w375, 7:w275, 8:w377, 11:w378) -> (0:w370:errorcluster, 3:w374:refnum<k34>)  [unwired: 2 in, 2 out]
  n138 = call <vilib>:"Simple Error Handler.vi"("error source (\" \")"="Error in creating .tdms notes" ("error source (\" \")"), "error in (no error)"=w370) -> ()  [unwired: 3 in, 5 out]
  n139 = TDMS Open(6:FALSE ("disable buffering? (T)"), 7:enum16{"1.0", "2.0"}."1.0" ("file format version (2.0)"), 10:T5."create" ("operation (0:open)"), 11:w120) -> (3:w123:refnum<k34>)  [unwired: 3 in, 1 out]
  n140 = call-poly <vilib>:"DAQmx Write.vi"("task/channels in"=w316, "data"=TRUE, "error in"=w317) -> ("task out"=w314:refnum<k21>, "error out"=w312:errorcluster)  [unwired: 10 in, 1 out]
  n141 = case shown="True" "LED" {
    tunnel: [w707 w714] -> w37
    tunnel: [w706 w713] -> w36
    tunnel: w87 -> [w707 w712]
    tunnel: w86 -> [w706 w711]
    tunnel: w85 -> [_ w708]
    frame False {
    }
    frame True {
      n142 = call-poly <vilib>:"DAQmx Write.vi"("task/channels in"=w712, "data"=w708, "error in"=w711) -> ("task out"=w709:refnum<k21>, "error out"=w715:errorcluster)  [unwired: 10 in, 1 out]
      n143 = First Call?() -> (First Call?: T/F=w710:bool)
      n144 = case shown="True" w710 {
        tunnel: w709 -> [w716 w721]
        tunnel: w715 -> [w717 w720]
        tunnel: [w716 w719] -> w714
        tunnel: [w717 w718] -> w713
        frame False {
        }
        frame True {
          n145 = call <vilib>:"DAQmx Start Task.vi"("task/channels in"=w721, "error in"=w720) -> ("task out"=w719:refnum<k21>, "error out"=w718:errorcluster)  [unwired: 12 in]
        }
      }
    }
  }
  n146 = while {
    tunnel: w458 -> [w789]
    tunnel: w456 -> [w790]
    tunnel: [w770] -> w502
    tunnel: [w768] -> w503
    tunnel: [w784] -> w501
    tunnel: [w779] -> w454
    tunnel: w453 -> [w779]
    tunnel: [w778] -> w452
    tunnel: w451 -> [w778]
    tunnel: w450 -> [w777]
    tunnel: w448 -> [w776]
    tunnel: w447 -> [w775]
    tunnel: w445 -> [w767]
    tunnel: w314 -> [w772]
    tunnel: [w772] -> w313
    tunnel: [w771] -> w311
    tunnel: w312 -> [w771]
    tunnel: w118 -> [w762]
    tunnel: [w746] -> w72
    tunnel: [w747] -> w71
    tunnel: [w748] -> w70
    tunnel: [w749] -> w69
    tunnel: [w750] -> w68
    tunnel: [w751] -> w67
    tunnel: w66 -> [w752]
    tunnel: w65 -> [w753]
    tunnel: w64 -> [w754]
    tunnel: w63 -> [w755]
    tunnel: w62 -> [w756]
    tunnel: w61 -> [w757]
    tunnel: "Solenoids" -> [w758]
    tunnel: w47 -> [w744]
    tunnel: w44 -> [w743]
    tunnel: w41 -> [w742]
    tunnel: w38 -> [w741]
    tunnel: w3 -> [w727]
    i -> [w763]
    stop <- w740 stop-if-true
    n147 = Greater?(x=w763, y=w762) -> (0:→"CBV Cam":bool)
    n148 = call <vilib>:"IMAQ Extract Buffer.vi"("error in (no error)"=w790, "Buffer to extract"=w763, "IMAQ Session In"=w789) -> ("error out"=w783:errorcluster, "Buffer Number"=w745:i32, "Image Out"=w760:T1, "IMAQ Session Out"=w768:refnum<k11>)  [unwired: 5 out]
    "Last CBV\nBuffer" <- w745
    "?" <- w760
    n149 = Multiply(x=w744, y=w745) -> (x*y=w759:dbl)
    n150 = Round Toward -Infinity(1:w759) -> (0:w726:dbl)
    n151 = Tick Count (ms)() -> (millisecond timer value=w782:u32)
    n152 = call <vilib>:"Calculate Frames per Second.vi"("Update Interval (ms)"=u32 2000, "Buffer Number"=w745) -> ("Processed Frames/s"=→"CBV Cam":dbl)  [unwired: 7 in, 2 out]
    n153 = Index Array(array=w743, index (row)=w726) -> (element=w737:bool[])  [unwired: 1 in]
    n154 = Index Array(array=w742, index (row)=w726) -> (element=w733:bool[])  [unwired: 1 in]
    n155 = Index Array(array=w741, index (row)=w726) -> (element=w734:bool[])  [unwired: 1 in]
    n156 = Index Array(array=w727, index (row)=w726) -> (element=w728:bool[])  [unwired: 1 in]
    n157 = Greater Or Equal?(x=w745, y=w776) -> (x >= y?=w766:bool)
    n158 = call "IMAQ ImageToArray"("error in (no error)"=w783, "Image"=w760) -> ("error out"=w788:errorcluster, "Image Pixels (I16)"=w787:i16[][])  [unwired: 2 in, 3 out]
    n159 = Subtract(x=w782, y=w777) -> (x-y=w781:u32)
    n160 = local write "stop"("stop") -> ()
    n161 = case shown="True" w758 {
      tunnel: w753 -> [w792 w811]
      tunnel: w752 -> [w791 w810]
      tunnel: [w792 w809] -> w750
      tunnel: [w791 w808] -> w751
      tunnel: w755 -> [w794 w807]
      tunnel: w754 -> [w793 w806]
      tunnel: [w794 w805] -> w748
      tunnel: [w793 w804] -> w749
      tunnel: w757 -> [w796 w803]
      tunnel: w756 -> [w795 w802]
      tunnel: [w796 w801] -> w746
      tunnel: [w795 w800] -> w747
      tunnel: w737 -> [_ w799]
      tunnel: w733 -> [_ w798]
      tunnel: w734 -> [_ w797]
      frame False {
      }
      frame True {
        n162 = call-poly <vilib>:"DAQmx Write.vi"("task/channels in"=w803, "data"=w799, "error in"=w802) -> ("task out"=w801:refnum<k21>, "error out"=w800:errorcluster)  [unwired: 10 in, 1 out]
        n163 = call-poly <vilib>:"DAQmx Write.vi"("task/channels in"=w807, "data"=w798, "error in"=w806) -> ("task out"=w805:refnum<k21>, "error out"=w804:errorcluster)  [unwired: 10 in, 1 out]
        n164 = call-poly <vilib>:"DAQmx Write.vi"("task/channels in"=w811, "data"=w797, "error in"=w810) -> ("task out"=w809:refnum<k21>, "error out"=w808:errorcluster)  [unwired: 10 in, 1 out]
      }
    }
    n165 = Greater?(x=w737, y=FALSE ("Boolean")) -> (0:w738:bool[])
    n166 = Greater?(x=w733, y=FALSE ("Boolean")) -> (0:w735:bool[])
    n167 = Greater?(x=w734, y=FALSE ("Boolean")) -> (0:w736:bool[])
    n168 = Greater?(x=w728, y=FALSE ("Boolean")) -> (0:w729:bool[])
    n169 = Multiply(x=w781, y=1.667e-05) -> (x*y=w780:dbl)
    n170 = Or Array Elements(Boolean array=w738) -> (logical OR=→"LPad":bool)
    n171 = Or Array Elements(Boolean array=w735) -> (logical OR=→"Auditory":bool)
    n172 = Or Array Elements(Boolean array=w736) -> (logical OR=→"RPad":bool)
    n173 = Or Array Elements(Boolean array=w729) -> (logical OR=→"LED":bool)
    n174 = Write to Binary File(file (use dialog)=w767, data=w787, error in=w788, 5:FALSE ("prepend array or string size? (T)"), 9:T11."big-endian, network order" ("byte order (0:big-endian, network order)")) -> (refnum out=w784:refnum<file>, error out=w770:errorcluster)  [unwired: 1 in, 1 out]
    n175 = Bundle("Time (min)"=w775, w780) -> (→"Time Elapsed (Min)":cluster{"Time (min)":dbl, dbl})  [unwired: 1 in]
    n176 = Compound Arithmetic op=OR(w770, w766, "stop") -> (w740:bool)
    "CBV Camera" <- w740
    "Finished" <- w740
  }
  n177 = while {
    tunnel: w231 -> [w837]
    tunnel: [w838] -> w197
    tunnel: w230 -> [w838]
    tunnel: [w837] -> w196
    tunnel: [w826] -> w194
    tunnel: [w827] -> w195
    tunnel: [w836] -> w193
    tunnel: w229 -> [w835]
    tunnel: w228 -> [w834]
    tunnel: w222 -> [w833]
    tunnel: w227 -> [w832]
    shift-right: [w825] -> _
    shift-left: _ -> [w831]
    shift-right: [w830] -> _
    shift-left: u32 0 ("New Lost") -> [w824]
    shift-right: [w829] -> w191
    shift-left: u32[] [] ("NewBuffNum") -> [w820]
    shift-right: [w828] -> w192
    shift-left: u32[] [] ("NewNumLost") -> [w821]
    tunnel: w212 -> [w819]
    tunnel: w118 -> [w816]
    i -> [w817]
    stop <- w822 stop-if-true
    n178 = call <vilib>:"IMAQdx Get Image.vi"("Buffer Number Mode (Next)"=IMAQdx_Buffer_Number_Mode."Next", "error in"=w834, "Image In"=w833, "Session In"=w835) -> ("error out"=w845:errorcluster, "Buffer Number Out"=w825:u32, "Image Out"=w813:T1, "Session Out"=w826:T4)  [unwired: 4 in]
    "Last Whisk\nBuffer 2" <- w825
    "?" <- w813
    n179 = Greater?(x=w817, y=w816) -> (0:→"Pupil Cam":bool)
    n180 = call "TrackPupilDroppedFrames_IOS.vi"("NumLost"=w821, "BuffNum"=w820, "Curr Buffer"=w825, "Prev Lost"=w824, "Prev Buffer"=w831) -> ("New Lost"=w830:u32, "NewNumLost"=w828:u32[], "NewBuffNum"=w829:u32[])  [unwired: 4 in]
    "Dropped 2" <- w830
    n181 = call "IMAQ ImageToArray"("error in (no error)"=w845, "Image"=w813) -> ("error out"=w844:errorcluster, "Image Pixels (U8)"=w843:u8[][])  [unwired: 2 in, 3 out]
    n182 = Add(x=w825, y=w824) -> (x+y=w823:u32)
    n183 = Greater Or Equal?(x=w823, y=w819) -> ()  [unwired: 1 out]
    n184 = Write to Binary File(file (use dialog)=w832, data=w843, error in=w844, 5:FALSE ("prepend array or string size? (T)"), 9:T11."little-endian" ("byte order (0:big-endian, network order)")) -> (refnum out=w836:refnum<file>, error out=w827:errorcluster)  [unwired: 1 in, 1 out]
    n185 = local read "stop"() -> (w815:bool)
    n186 = local read "CBV Camera"() -> (w814:bool)
    n187 = call <vilib>:"Calculate Frames per Second.vi"("Update Interval (ms)"=u32 2000, "Buffer Number"=w825) -> ("Processed Frames/s"=→"Pupil Cam Fs":dbl)  [unwired: 7 in, 2 out]
    n188 = Unbundle By Name(w827) -> ("status"=w812:bool)
    n189 = Compound Arithmetic op=OR(w812, w815, w814) -> (w822:bool)
  }
  n190 = while {
    tunnel: w474 -> [w873]
    tunnel: [w874] -> w473
    tunnel: w472 -> [w874]
    tunnel: [w873] -> w471
    tunnel: [w866] -> w334
    tunnel: [w867] -> w391
    tunnel: [w872] -> w470
    tunnel: w469 -> [w871]
    tunnel: w467 -> [w870]
    tunnel: w465 -> [w869]
    tunnel: w463 -> [w868]
    shift-right: [w856] -> _
    shift-left: _ -> [w854]
    shift-right: [w851] -> _
    shift-left: u32 0 ("New Lost") -> [w855]
    shift-right: [w852] -> w326
    shift-left: u32[] [] ("NewBuffNum") -> [w853]
    shift-right: [w858] -> w415
    shift-left: u32[] [] ("NewNumLost") -> [w857]
    tunnel: w213 -> [w864]
    tunnel: w118 -> [w859]
    i -> [w860]
    stop <- w863 stop-if-true
    n191 = call <vilib>:"IMAQdx Get Image.vi"("Buffer Number Mode (Next)"=IMAQdx_Buffer_Number_Mode."Next", "error in"=w870, "Image In"=w869, "Session In"=w871) -> ("error out"=w880:errorcluster, "Buffer Number Out"=w856:u32, "Image Out"=w848:T1, "Session Out"=w866:T4)  [unwired: 4 in]
    "Last Whisk\nBuffer" <- w856
    "?" <- w848
    n192 = Greater?(x=w860, y=w859) -> (0:→"Whisk Cam":bool)
    n193 = call "IMAQ ImageToArray"("error in (no error)"=w880, "Image"=w848) -> ("error out"=w879:errorcluster, "Image Pixels (U8)"=w878:u8[][])  [unwired: 2 in, 3 out]
    n194 = call "TrackWhiskDroppedFrames_IOS.vi"("NumLost"=w857, "BuffNum"=w853, "Curr Buffer"=w856, "Prev Lost"=w855, "Prev Buffer"=w854) -> ("New Lost"=w851:u32, "NewNumLost"=w858:u32[], "NewBuffNum"=w852:u32[])  [unwired: 4 in]
    "Dropped" <- w851
    n195 = Add(x=w856, y=w855) -> (x+y=w865:u32)
    n196 = Greater Or Equal?(x=w865, y=w864) -> ()  [unwired: 1 out]
    n197 = Write to Binary File(file (use dialog)=w868, data=w878, error in=w879, 5:FALSE ("prepend array or string size? (T)"), 9:T11."little-endian" ("byte order (0:big-endian, network order)")) -> (refnum out=w872:refnum<file>, error out=w867:errorcluster)  [unwired: 1 in, 1 out]
    n198 = local read "stop"() -> (w850:bool)
    n199 = local read "CBV Camera"() -> (w849:bool)
    n200 = call <vilib>:"Calculate Frames per Second.vi"("Update Interval (ms)"=u32 2000, "Buffer Number"=w856) -> ("Processed Frames/s"=→"Whisk Cam Fs":dbl)  [unwired: 7 in, 2 out]
    n201 = Unbundle By Name(w867) -> ("status"=w847:bool)
    n202 = Compound Arithmetic op=OR(w847, w850, w849) -> (w863:bool)
  }
  n203 = while {
    tunnel: w490 -> [w898]
    tunnel: w484 -> [w896]
    tunnel: w482 -> [w895]
    tunnel: w480 -> [w894]
    tunnel: w477 -> [w892]
    tunnel: [w893] -> w226
    tunnel: [w884] -> w475
    tunnel: [w892] -> w476
    tunnel: w118 -> [w887]
    i -> [w888]
    stop <- w885 stop-if-true
    n204 = Tick Count (ms)() -> (millisecond timer value=w900:u32)
    n205 = Subtract(x=w900, y=w898) -> (x-y=w901:u32)
    n206 = Divide(x=w901, y=u32 1000) -> (x/y=w897:dbl)
    n207 = Greater?(x=w888, y=w887) -> (0:→"Web Cam":bool)
    n208 = call "GrabWebCam_IOS.vi"("Session In"=w895, "Image In"=w896, "Trial Time"=w897, "AVI Refnum"=w892, "error in"=w894) -> ("Session Out"=w893:T4, "WebCam Img Out"=→"?":T1, "Buffer Number Out"=w891:u32, "error out"=w884:errorcluster)  [unwired: 7 in]
    n209 = local read "CBV Camera"() -> (w886:bool)
    n210 = local read "stop"() -> (w883:bool)
    n211 = call <vilib>:"Calculate Frames per Second.vi"("Update Interval (ms)"=u32 5000, "Buffer Number"=w891) -> ("Processed Frames/s"=→"Web Cam Fs":dbl)  [unwired: 7 in, 2 out]
    n212 = Compound Arithmetic op=OR(w884, w883, w886) -> (w885:bool)
  }
  n213 = while {
    tunnel: w433 -> [w925]
    tunnel: w432 -> [w924]
    tunnel: w146 -> [w923]
    tunnel: [w922] -> w186
    tunnel: [w911] -> w185
    tunnel: [w921] -> w429
    shift-right: [w915] -> _
    shift-left: w118 -> [w906]
    tunnel: [w911] -> w276
    tunnel: w147 -> [w909]
    i -> [w907]
    stop <- w912 stop-if-true
    n214 = To Long Integer(number=w909) -> (32bit integer=w910:i32)
    n215 = call-poly <vilib>:"DAQmx Read.vi"("task/channels in"=w924, "error in"=w925) -> ("task out"=w921:refnum<k21>, "data"=w903:waveform(dbl)[], "error out"=w914:errorcluster)  [unwired: 11 in]
    n216 = Greater?(x=w906, y=w907) -> (0:→"Dev1 Analog":bool)
    n217 = TDMS Write(0:w923, 5:"Analog Data" ("group name in (Untitled)"), 9:w903, 11:w914) -> (4:w922:refnum<k34>, 15:w911:errorcluster)  [unwired: 2 in, 2 out]
    n218 = Index Array(array=w903, index=0) -> (element=w918:waveform(dbl))
    n219 = Unbundle By Name(w918) -> ("Y"=w917:dbl[])
    n220 = local read "CBV Camera"() -> (w905:bool)
    n221 = local read "stop"() -> (w904:bool)
    n222 = Array Size(array=w917) -> (size(s)=w916:i32)
    n223 = Add(x=w916, y=w906) -> (x+y=w915:i32)
    "Dev1 Samples" <- w915
    n224 = Greater Or Equal?(x=w915, y=w910) -> (x >= y?=w913:bool)
    n225 = Compound Arithmetic op=OR(w911, w913, w904, w905) -> (w912:bool)
  }
  n226 = while {
    tunnel: w144 -> [w948]
    tunnel: w145 -> [w947]
    tunnel: [w946] -> w130
    tunnel: [w935] -> w131
    tunnel: [w945] -> w141
    shift-right: [w939] -> _
    shift-left: w118 -> [w930]
    tunnel: [w935] -> w140
    tunnel: w147 -> [w933]
    tunnel: w121 -> [w927]
    i -> [w931]
    stop <- w936 stop-if-true
    n227 = To Long Integer(number=w933) -> (32bit integer=w934:i32)
    n228 = call-poly <vilib>:"DAQmx Read.vi"("task/channels in"=w947, "error in"=w948) -> ("task out"=w945:refnum<k21>, "data"=w926:waveform(dbl)[], "error out"=w938:errorcluster)  [unwired: 11 in]
    n229 = Greater?(x=w930, y=w931) -> (0:→"Dev2 Analog":bool)
    n230 = TDMS Write(0:w927, 5:"Analog Data" ("group name in (Untitled)"), 9:w926, 11:w938) -> (4:w946:refnum<k34>, 15:w935:errorcluster)  [unwired: 2 in, 2 out]
    n231 = Index Array(array=w926, index=0) -> (element=w942:waveform(dbl))
    n232 = Unbundle By Name(w942) -> ("Y"=w941:dbl[])
    n233 = local read "CBV Camera"() -> (w929:bool)
    n234 = local read "stop"() -> (w928:bool)
    n235 = Array Size(array=w941) -> (size(s)=w940:i32)
    n236 = Add(x=w940, y=w930) -> (x+y=w939:i32)
    "Dev2 Samples" <- w939
    n237 = Greater Or Equal?(x=w939, y=w934) -> (x >= y?=w937:bool)
    n238 = Compound Arithmetic op=OR(w935, w937, w928, w929) -> (w936:bool)
  }
  n239 = while {
    tunnel: [w951] -> w35
    tunnel: w37 -> [w951]
    tunnel: w36 -> [w950]
    tunnel: [w950] -> w34
    stop <- w949 stop-if-true
    n240 = local read "Finished"() -> (w949:bool)
  }
  n241 = call <vilib>:"DAQmx Stop Task.vi"("task/channels in"=w141, "error in"=w140) -> ("task out"=w143:refnum<k21>, "error out"=w142:errorcluster)  [unwired: 12 in]
  n242 = call <vilib>:"DAQmx Stop Task.vi"("task/channels in"=w429, "error in"=w276) -> ("task out"=w393:refnum<k21>, "error out"=w392:errorcluster)  [unwired: 12 in]
  n243 = call <vilib>:"IMAQ Extract Buffer.vi"("error in (no error)"=w502, "Buffer to extract"=-1, "IMAQ Session In"=w503) -> ("error out"=w524:errorcluster, "IMAQ Session Out"=w523:refnum<k11>)  [unwired: 7 out]
  n244 = Close File(refnum=w501, error in=w185) -> (path=w409:path)  [unwired: 1 out]
  n245 = Delete From Array(array=w326, length=1, index=0) -> (array with subset deleted=w288:u32[])  [unwired: 1 out]
  n246 = call-poly <vilib>:"DAQmx Write.vi"("task/channels in"=w313, "data"=FALSE, "error in"=w311) -> ("task out"=w310:refnum<k21>, "error out"=w308:errorcluster)  [unwired: 10 in, 1 out]
  n247 = Delete From Array(array=w415, length=1, index=0) -> (array with subset deleted=w289:u32[])  [unwired: 1 out]
  n248 = call <vilib>:"DAQmx Stop Task.vi"("task/channels in"=w196, "error in"=w197) -> ("task out"=w177:refnum<k21>, "error out"=w178:errorcluster)  [unwired: 12 in]
  n249 = call <vilib>:"DAQmx Stop Task.vi"("task/channels in"=w471, "error in"=w473) -> ("task out"=w175:refnum<k21>, "error out"=w176:errorcluster)  [unwired: 12 in]
  n250 = Delete From Array(array=w192, length=1, index=0) -> (array with subset deleted=w199:u32[])  [unwired: 1 out]
  n251 = Delete From Array(array=w191, length=1, index=0) -> (array with subset deleted=w198:u32[])  [unwired: 1 out]
  n252 = call <vilib>:"IMAQdx Close Camera.vi"("error in"=w391, "Session In"=w334) -> ()  [unwired: 9 in, 1 out]
  n253 = Close File(refnum=w470, error in=w391) -> (path=w407:path, error out=w406:errorcluster)
  n254 = call "IMAQ AVI2 Close"("error in (no error)"=w475, "AVI Refnum"=w476) -> ("error out"=w408:errorcluster)  [unwired: 9 in]
  n255 = call <vilib>:"IMAQdx Close Camera.vi"("error in"=w475, "Session In"=w226) -> ()  [unwired: 9 in, 1 out]
  n256 = call <vilib>:"DAQmx Clear Task.vi"("task in"=w143, "error in"=w142) -> ()  [unwired: 13 in, 1 out]
  n257 = call <vilib>:"IMAQdx Close Camera.vi"("error in"=w195, "Session In"=w194) -> ()  [unwired: 9 in, 1 out]
  n258 = Close File(refnum=w193, error in=w195) -> (path=w188:path, error out=w187:errorcluster)
  n259 = Build Array(w288, w289) -> (w291:u32[][])
  n260 = call <vilib>:"DAQmx Clear Task.vi"("task in"=w393, "error in"=w392) -> ()  [unwired: 13 in, 1 out]
  n261 = call <vilib>:"DAQmx Stop Task.vi"("task/channels in"=w35, "error in"=w34) -> ("task out"=w97:refnum<k21>, "error out"=w96:errorcluster)  [unwired: 12 in]
  n262 = call <vilib>:"DAQmx Stop Task.vi"("task/channels in"=w310, "error in"=w308) -> ("task out"=w309:refnum<k21>, "error out"=w307:errorcluster)  [unwired: 12 in]
  n263 = call <vilib>:"DAQmx Stop Task.vi"("task/channels in"=w72, "error in"=w71) -> ("task out"=w74:refnum<k21>, "error out"=w73:errorcluster)  [unwired: 12 in]
  n264 = call <vilib>:"DAQmx Stop Task.vi"("task/channels in"=w70, "error in"=w69) -> ("task out"=w76:refnum<k21>, "error out"=w75:errorcluster)  [unwired: 12 in]
  n265 = call <vilib>:"DAQmx Stop Task.vi"("task/channels in"=w68, "error in"=w67) -> ("task out"=w78:refnum<k21>, "error out"=w77:errorcluster)  [unwired: 12 in]
  n266 = call <vilib>:"DAQmx Stop Task.vi"("task/channels in"=w454, "error in"=w452) -> ("task out"=w179:refnum<k21>, "error out"=w180:errorcluster)  [unwired: 12 in]
  n267 = call <vilib>:"IMAQ Close.vi"("error in (no error)"=w524, "IMAQ Session In"=w523) -> ("error out"=w525:errorcluster)  [unwired: 9 out]
  n268 = Build Array(w198, w199) -> (w201:u32[][])
  n269 = call <vilib>:"DAQmx Clear Task.vi"("task in"=w175, "error in"=w176) -> ()  [unwired: 13 in, 1 out]
  n270 = call <vilib>:"DAQmx Clear Task.vi"("task in"=w177, "error in"=w178) -> ()  [unwired: 13 in, 1 out]
  n271 = Array To Spreadsheet String(delimiter (Tab)=",", array=w289, 3:"%d" ("format string")) -> (spreadsheet string=w327:string)
  n272 = Transpose 2D Array(2D array=w291) -> (transposed array=w290:u32[][])
  n273 = Array To Spreadsheet String(delimiter (Tab)=",", array=w288, 3:"%d" ("format string")) -> (spreadsheet string=w328:string)
  n274 = Move(source path=w188, error in=w187, 10:"Target Path") -> (error out=w189:errorcluster)  [unwired: 2 in, 2 out]
  n275 = Move(source path=w407, error in=w406, 10:"Target Path") -> (error out=w404:errorcluster)  [unwired: 2 in, 2 out]
  n276 = Array To Spreadsheet String(delimiter (Tab)=",", array=w199, 3:"%d" ("format string")) -> (spreadsheet string=w202:string)
  n277 = Transpose 2D Array(2D array=w201) -> (transposed array=w200:u32[][])
  n278 = Array To Spreadsheet String(delimiter (Tab)=",", array=w198, 3:"%d" ("format string")) -> (spreadsheet string=w203:string)
  n279 = Move(source path=w31, error in=w408, 10:"Target Path") -> (error out=w403:errorcluster)  [unwired: 2 in, 2 out]
  n280 = call <vilib>:"DAQmx Clear Task.vi"("task in"=w74, "error in"=w73) -> ()  [unwired: 13 in, 1 out]
  n281 = call <vilib>:"DAQmx Clear Task.vi"("task in"=w76, "error in"=w75) -> ()  [unwired: 13 in, 1 out]
  n282 = call <vilib>:"DAQmx Clear Task.vi"("task in"=w78, "error in"=w77) -> ()  [unwired: 13 in, 1 out]
  n283 = call <vilib>:"DAQmx Clear Task.vi"("task in"=w179, "error in"=w180) -> ()  [unwired: 13 in, 1 out]
  n284 = TDMS Close(8:w131, 11:w130) -> (0:w139:errorcluster, 3:w119:path)
  n285 = call <vilib>:"DAQmx Clear Task.vi"("task in"=w97, "error in"=w96) -> ()  [unwired: 13 in, 1 out]
  n286 = call <vilib>:"DAQmx Clear Task.vi"("task in"=w309, "error in"=w307) -> ()  [unwired: 13 in, 1 out]
  n287 = for {
    N: w278 -> [_]
    tunnel: w519 -> [w955] mode=indexing
    shift-right: [w953] -> w411
    shift-left: w525 -> [w954]
    n288 = call "IMAQ Dispose"("All Images? (No)"=FALSE, "Image"=w955, "error in (no error)"=w954) -> ("error out"=w953:errorcluster)  [unwired: 3 out]
  }
  n289 = call <vilib>:"Trim Whitespace.vi"("string"=w328) -> ("trimmed string"=w171:string)  [unwired: 1 in]
  n290 = call <vilib>:"Trim Whitespace.vi"("string"=w327) -> ("trimmed string"=w170:string)  [unwired: 1 in]
  n291 = Number To Decimal String(number=w290) -> ()  [unwired: 1 in, 1 out]
  n292 = call <vilib>:"Trim Whitespace.vi"("string"=w203) -> ("trimmed string"=w172:string)  [unwired: 1 in]
  n293 = call <vilib>:"Trim Whitespace.vi"("string"=w202) -> ("trimmed string"=w173:string)  [unwired: 1 in]
  n294 = Number To Decimal String(number=w200) -> ()  [unwired: 1 in, 1 out]
  n295 = call <vilib>:"Simple Error Handler.vi"("error in (no error)"=w189) -> ()  [unwired: 1 in, 8 out]
  n296 = call <vilib>:"Simple Error Handler.vi"("error in (no error)"=w404) -> ()  [unwired: 1 in, 8 out]
  n297 = Path To String(path=w119) -> (string=w137:string)
  n298 = call <vilib>:"Simple Error Handler.vi"("error in (no error)"=w403) -> ()  [unwired: 1 in, 8 out]
  n299 = TDMS Defragment(4:w139, 7:w119) -> (0:w133:errorcluster)
  n300 = Build Array(w172, w173, w171, w170) -> (w169:string[])
  n301 = Concatenate Strings(w137, "_index" ("string")) -> (w135:string)
  n302 = Move(source path=w409, error in=w411, 10:"Target Path") -> (error out=w410:errorcluster)  [unwired: 2 in, 2 out]
  n303 = String To Path(string=w135) -> (path=w134:path)
  n304 = call <vilib>:"Simple Error Handler.vi"("error in (no error)"=w410) -> ()  [unwired: 1 in, 8 out]
  n305 = Move(source path=w119, error in=w133, 10:"Target Path") -> (error out=w138:errorcluster)  [unwired: 2 in, 2 out]
  n306 = Move(source path=w134, error in=w133, 10:"Target Path") -> (error out=w132:errorcluster)  [unwired: 2 in, 2 out]
  n307 = TDMS Set Properties(5:w169, 7:string[] ["PupilCam_DroppedFrameIndex", "PupilCam_NumberDropped", "WhiskCam_DroppedFrameIndex", "WhiskCam_NumberDropped"] ("channel name(s) in (Untitled)"), 8:w185, 11:w186) -> (0:w335:errorcluster, 3:w333:refnum<k34>)  [unwired: 2 in, 2 out]
  n308 = call <vilib>:"Simple Error Handler.vi"("error in (no error)"=w138) -> ()  [unwired: 1 in, 8 out]
  n309 = call <vilib>:"Simple Error Handler.vi"("error in (no error)"=w132) -> ()  [unwired: 1 in, 8 out]
  n310 = TDMS Close(8:w335, 11:w333) -> (0:w412:errorcluster, 3:w400:path)
  n311 = Path To String(path=w400) -> (string=w402:string)
  n312 = TDMS Defragment(4:w412, 7:w400) -> (0:w397:errorcluster)
  n313 = Concatenate Strings(w402, "_index" ("string")) -> (w399:string)
  n314 = String To Path(string=w399) -> (path=w398:path)
  n315 = Move(source path=w400, error in=w397, 10:"Target Path") -> (error out=w405:errorcluster)  [unwired: 2 in, 2 out]
  n316 = Move(source path=w398, error in=w397, 10:"Target Path") -> (error out=w190:errorcluster)  [unwired: 2 in, 2 out]
  n317 = call <vilib>:"Simple Error Handler.vi"("error in (no error)"=w405) -> ()  [unwired: 1 in, 8 out]
  n318 = call <vilib>:"Simple Error Handler.vi"("error in (no error)"=w190) -> ()  [unwired: 1 in, 8 out]
